vi "Add (bytes).vi"(9 "value":u8[](array[numeric]), 10 "key":u8[](array[numeric]), 11 "MsgPackMap in":refnum<class "MsgPackMap.lvclass">) -> (3 "MsgPackMap out":refnum<class "MsgPackMap.lvclass">)   [LabVIEW 2020, in "MessagePack.lvlib" / "MsgPackMap.lvclass"]
uses:
  MsgPackMap.lvclass
  MsgPackMap.lvclass/MsgPackMap.ctl
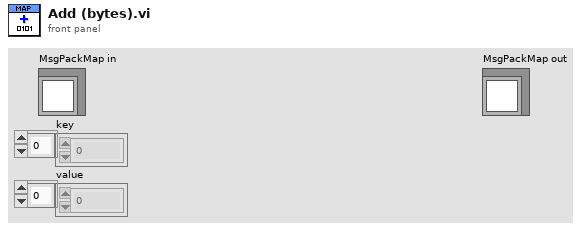
[diagram p1: front panel]
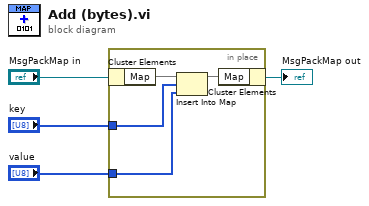
[diagram p0: block diagram]
diagram:
  n1 = in-place {
    in-place-border: "key" -> [w7]
    in-place-border: "value" -> [w6]
    n2 = in-place-cluster #1("MsgPackMap in") -> ("Map"=w8:map{u8[], u8[]})
    n3 = Insert Into Map(map in=w8, key=w7, value=w6) -> (map out=w5:map{u8[], u8[]})  [unwired: 2 out]
    n4 = in-place-cluster #1("Map"=w5) -> (→"MsgPackMap out":refnum<class "MsgPackMap.lvclass">)
  }
